vi "Synthesize.vi"(6 "last":bool, 8 "error in (no error)":errorcluster, 9 "Repetition":i32, 11 "SigMan in":refnum<class "SignalManager.lvclass">) -> (0 "error out":errorcluster, 2 "Array":dbl[][](array[numeric]), 3 "SigMan out":refnum<class "SignalManager.lvclass">)   [LabVIEW 2020, in "SignalManager.lvclass"]
uses:
  SignalManager.lvclass
  Channel/Channel.lvclass
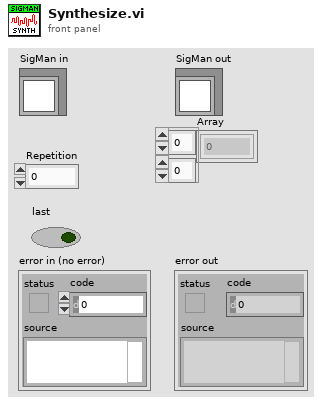
[diagram p1: front panel]
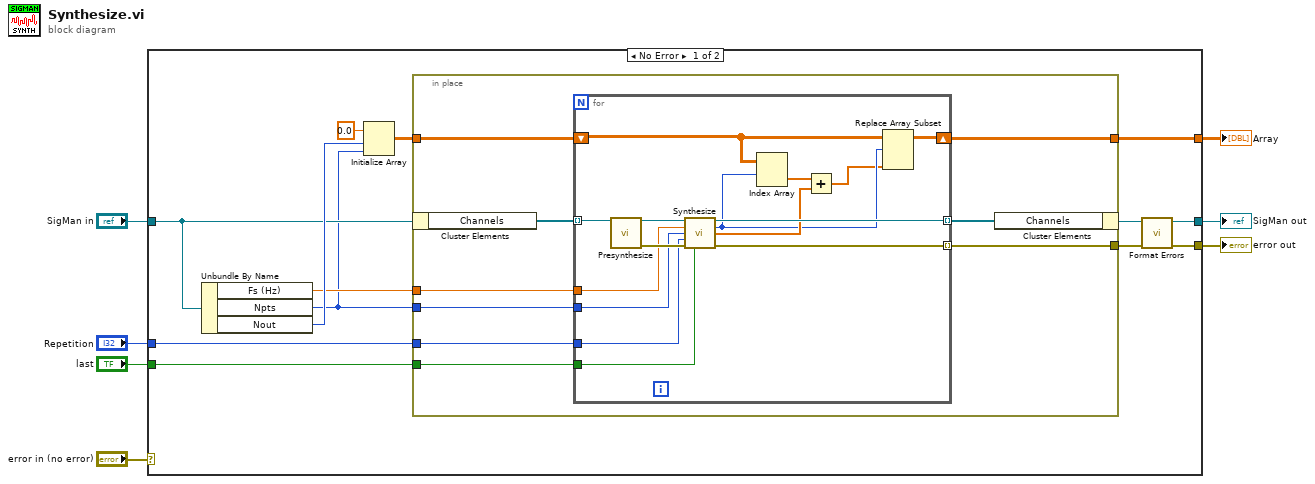
[diagram p0: block diagram]
diagram:
  n1 = case shown="No Error" "error in (no error)" {
    selector: "error in (no error)" -> [_ w46]
    tunnel: [w9 w46] -> w6
    tunnel: [w10 w45] -> w4
    tunnel: "SigMan in" -> [w18 w45]
    tunnel: "Repetition" -> [w15 _]
    tunnel: [w13 _] -> w2
    tunnel: "last" -> [w8 _]
    frame No Error {
      n2 = Unbundle By Name(w18) -> ("Fs (Hz)"=w17:dbl, "Npts"=w16:i32, "Nout"=w20:i32)
      n3 = Initialize Array(0.0 ("element"), w20, w16) -> (w14:dbl[][])
      n4 = in-place {
        in-place-border: w17 -> [w28]
        in-place-border: w16 -> [w27]
        in-place-border: w15 -> [w26]
        in-place-border: w14 -> [w25]
        in-place-border: [w23] -> w13
        in-place-border: [w22] -> w11
        in-place-border: w8 -> [w21]
        n5 = in-place-cluster #1(w18) -> ("Channels"=w29:refnum<class "Channel.lvclass">[])
        n6 = for {
          tunnel: w29 -> [w33] mode=indexing
          tunnel: w28 -> [w43]
          tunnel: w27 -> [w42]
          tunnel: w26 -> [w41]
          shift-right: [w36] -> w23
          shift-left: w25 -> [w37]
          tunnel: [w40] -> w24 mode=indexing
          tunnel: [w31] -> w22 mode=indexing
          tunnel: w21 -> [w30]
          n7 = call "Presynthesize.vi"("Channel in"=w33) -> ("Channel out"=w32:refnum<class "Channel.lvclass">, "error out"=w44:errorcluster)  [unwired: 13 in]
          n8 = call "Synthesize.vi"("Channel in"=w32, "Fs (Hz)"=w43, "Npts"=w42, "Repetition"=w41, "error in (no error)"=w44, "last"=w30) -> ("Channel out"=w40:refnum<class "Channel.lvclass">, "Number"=w35:i32, "Array"=w38:dbl[], "error out"=w31:errorcluster)  [unwired: 6 in]
          n9 = Index Array(array=w37, index (row)=w35) -> (element=w39:dbl[])  [unwired: 1 in]
          n10 = Add(x=w39, y=w38) -> (x+y=w34:dbl[])
          n11 = Replace Array Subset(array=w37, new element=w34, index (row)=w35) -> (w36:dbl[][])  [unwired: 1 in]
        }
        n12 = in-place-cluster #1("Channels"=w24) -> (w12:refnum<class "SignalManager.lvclass">)
      }
      n13 = call "Format Errors.vi"("error in (no error)"=w11, "SigMan in"=w12) -> ("error out"=w9:errorcluster, "SigMan out"=w10:refnum<class "SignalManager.lvclass">)  [unwired: 8 in]
    }
    frame Error {
    }
  }
  "error out" <- w6
  "SigMan out" <- w4
  "Array" <- w2
